vi "Begin.vi"() -> (0 "error out 2":errorcluster)   [LabVIEW 2014]
doc: "Called before other user functions, this VI is expected to open initial I/O refnums, load in file data, and do all program initialization. Notice that the <B>error out</B> terminal is simply used for data flow. Wiring it to other structures or subVIs ensures that this VI runs first."
uses:
  <vilib>/Rock Robotics/WPI/SafetyOutput/WPI_SafetyOutputConfigMenu.ctl
  <vilib>/Rock Robotics/WPI/DriverStation/WPI_DriverStationRobotMode2.ctl
  <vilib>/Rock Robotics/SystemInterfaces/DIO/FPGA_DIOPWMChannel.ctl
  <vilib>/Rock Robotics/WPI/Joystick/WPI_JoystickDeviceEnum.ctl
  <vilib>/Rock Robotics/SystemInterfaces/DIO/FPGA_DIOChannel.ctl
  <vilib>/Rock Robotics/SystemInterfaces/AI/FPGA_AIGyroChannel.ctl
  <vilib>/Rock Robotics/SystemInterfaces/Typedef/FPGA_TypedefAnalogModuleForGyro.ctl
  <vilib>/Rock Robotics/WPI/Solenoid/WPI_SolenoidChannel.ctl
  <vilib>/Rock Robotics/SystemInterfaces/Typedef/FPGA_TypedefDigitalModule.ctl
  <vilib>/Rock Robotics/SystemInterfaces/AI/FPGA_AIChannel.ctl
  <vilib>/Rock Robotics/SystemInterfaces/Typedef/FPGA_TypedefAnalogModule.ctl
  <vilib>/Rock Robotics/SystemInterfaces/DIO/FPGA_DIORelayChannel.ctl
  Robot Global Data.vi
  <vilib>/Rock Robotics/WPI/RobotDrive/WPI_RobotDriveOpen4MotorWithTalon.vi
  <vilib>/Rock Robotics/Network Tables/SD Write String Array.vi
  <vilib>/Rock Robotics/WPI/Counter/WPI_CounterDigitalInputToDigitalSource.vi
  <vilib>/Rock Robotics/WPI/Solenoid/WPI_SolenoidOpenDouble.vi
  <vilib>/Rock Robotics/WPI/Solenoid/WPI_SolenoidOpenSingle.vi
  <vilib>/Rock Robotics/WPI/MotorControl/WPI_MotorControlOpen Talon.vi
  TORC Code/GlobalVariable.vi
  Moose Code/Auto_Conf.vi
  <vilib>/Rock Robotics/WPI/Compressor/WPI_CompressorGetSetRefNum.vi
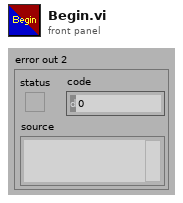
[diagram p1: front panel]
types:
  T1 = typedef "WPI_JoystickDeviceEnum.ctl" = enum16{"USB 0", "USB 1", "USB 2", "USB 3", "USB 4", "USB 5"}
  T2 = typedef "FPGA_DIORelayChannel.ctl" = enum8{"Relay 0", "Relay 1", "Relay 2", "Relay 3", "Invalid"}
  T3 = typedef "FPGA_DIOChannel.ctl" = enum8{"DIO 0", "DIO 1", "DIO 2", "DIO 3", "DIO 4", "DIO 5", "DIO 6", "DIO 7", "DIO 8", "DIO 9", "DIO MXP 0", "DIO MXP 1", "DIO MXP 2", "DIO MXP 3", "DIO MXP 4", "DIO MXP 5", "DIO MXP 6", "DIO MXP 7", "DIO MXP 8", "DIO MXP 9", "DIO MXP 10", "DIO MXP 11", "DIO MXP 12", "DIO MXP 13", "DIO MXP 14", "DIO MXP 15", "Invalid"}
  T4 = typedef "FPGA_TypedefAnalogModule.ctl" = enum16{"Controller 1"}
  T5 = typedef "FPGA_AIChannel.ctl" = enum8{"AI 0", "AI 1", "AI 2", "AI 3", "AI MXP 0", "AI MXP 1", "AI MXP 2", "AI MXP 3", "Invalid"}
  T6 = typedef "FPGA_DIOPWMChannel.ctl" = enum8{"PWM 0", "PWM 1", "PWM 2", "PWM 3", "PWM 4", "PWM 5", "PWM 6", "PWM 7", "PWM 8", "PWM 9", "PWM MXP 0", "PWM MXP 1", "PWM MXP 2", "PWM MXP 3", "PWM MXP 4", "PWM MXP 5", "PWM MXP 6", "PWM MXP 7", "PWM MXP 8", "PWM MXP 9", "Invalid"}
  T7 = typedef "FPGA_TypedefDigitalModule.ctl" = enum16{"Controller 1"}
  T8 = typedef "WPI_SolenoidChannel.ctl" = enum8{"Solenoid 0", "Solenoid 1", "Solenoid 2", "Solenoid 3", "Solenoid 4", "Solenoid 5", "Solenoid 6", "Solenoid 7", "Invalid"}
  T9 = typedef "FPGA_TypedefAnalogModuleForGyro.ctl" = enum16{"Controller 1"}
  T10 = typedef "FPGA_AIGyroChannel.ctl" = enum8{"AI 0", "AI 1", "Invalid"}
  T11 = typedef "WPI_DriverStationRobotMode2.ctl" = enum16{"Autonomous Disabled", "Autonomous Enabled", "Teleop Disabled", "Teleop Enabled", "Disconnected", "Finish", "Test Disabled", "Test Enabled", "Emergency Stopped"}
  T12 = typedef "WPI_SafetyOutputConfigMenu.ctl" = enum16{"Enable", "Disable"}
  T13 = typedef "WPI_JoystickDevRef.ctl" = cluster{"Device":T1}
  T14 = typedef "WPI_DigitalInputDevRef.ctl" = cluster{"DevStatus":errorcluster, "DIO Channel":T3, "Controller":T7}
  T15 = typedef "WPI_SolenoidDevRef.ctl" = cluster{"DevStatus":errorcluster, "Pneumatics Control Module":u8, "Forward Solenoid Channel":T8, "Reverse Solenoid Channel":T8}
  T16 = typedef "FPGA_CounterEncoderSourceConvertionLVSourceType.ctl" = cluster{"DevStatus":errorcluster, "AnalogTriggerMode?":bool, "DigitalMode":cluster{"Controller":T7, "DIO Channel":T17}, "AnalogTriggerMode":cluster{"AnalogTriggerIndex":T18, "OutputType":T19}}
  T17 = typedef "FPGA_DIODigitalSourceChannel.ctl" = enum8{"DIO 0", "DIO 1", "DIO 2", "DIO 3", "DIO 4", "DIO 5", "DIO 6", "DIO 7", "DIO 8", "DIO 9", "DIO MXP 0", "DIO MXP 1", "DIO MXP 2", "DIO MXP 3", "DIO MXP 4", "DIO MXP 5", "DIO MXP 6", "DIO MXP 7", "DIO MXP 8", "DIO MXP 9", "DIO MXP 10", "DIO MXP 11", "DIO MXP 12", "DIO MXP 13", "DIO MXP 14", "DIO MXP 15", "Disabled"}
  T18 = typedef "FPGA_AnalogTriggerIndex.ctl" = enum8{"Trig 0", "Trig 1", "Trig 2", "Trig 3", "Trig 4", "Trig 5", "Trig 6", "Trig 7", "Invalid"}
  T19 = typedef "FPGA_AnalogTriggerOutType.ctl" = enum16{"InWindow", "TriggerState", "Rising", "Falling"}
  T20 = typedef "WPI_RobotDriveDevRef.ctl" = cluster{"DevStatus":errorcluster, "Motors[]":T21[], "Square Inputs":bool, "Max Output":dbl}
  T21 = typedef "WPI_MotorControlDeviceRef.ctl" = cluster{"DeviceStatus":errorcluster, "Type":T22, "PWM":cluster{"Controller":T7, "PWM Channel":T6, "DeadBand":T23}, "CAN":cluster{"Device Number":u8, "Control Mode":T24, "Semaphore":T25, "Max Vout":dbl, "TalonSRX Control Mode":T26}, "Invert":bool, "TransformRef":T27, "InvTransformRef":T27}
  T22 = typedef "WPI_MotorControlType.ctl" = enum16{"PWM", "CAN", "CANTalonSRX"}
  T23 = typedef "WPI_PWMDeadband.ctl" = cluster{"Name":string, "maxPositivePwm":i32, "minPositivePwm":i32, "centerPwm":i32, "maxNegativePwm":i32, "minNegativePwm":i32, "angularRange":u16}
  T24 = typedef "WPI_CANJaguar_ControlMode.ctl" = enum8{"Percent VBus", "Current", "Speed", "Position", "Voltage"}
  T25 = typedef "Semaphore RefNum" = refnum<k1>
  T26 = typedef "WPI_CANTalonSRX_APIControlMode.ctl" = enum8{"Percent VBus", "Speed", "Position", "Slave", "Unchanged / Invalid"}
  T27 = typedef "WPI_PWMTransform_ConPane.ctl" = refnum<vi>
  T28 = typedef "WPI_EncoderDevRef.ctl" = cluster{"DevStatus":errorcluster, "EncoderIndex":T29, "CounterIndex":T30, "DistancePerCount":dbl, "Decoding Type":T31}
  T29 = typedef "FPGA_EncoderIdx.ctl" = enum8{"Enc 0", "Enc 1", "Enc 2", "Enc 3", "Enc 4", "Enc 5", "Enc 6", "Enc 7", "Invalid"}
  T30 = typedef "FPGA_CounterCtrSystemIndex.ctl" = enum8{"Ctr 0", "Ctr 1", "Ctr 2", "Ctr 3", "Ctr 4", "Ctr 5", "Ctr 6", "Ctr 7", "Invalid"}
  T31 = typedef "WPI_EncoderType.ctl" = enum16{"1x", "2x", "4x"}
  T32 = typedef "WPI_CompressorDevRef.ctl" = cluster{"DevStatus":errorcluster, "Pneumatics Control Module":u8}
  T33 = typedef "WPI_AnalogChannelDevRef.ctl" = cluster{"DevStatus":errorcluster, "Controller":T4, "Analog Channel":T5}
  T34 = typedef "WPI_RelayDevRef.ctl" = cluster{"DevStatus":errorcluster, "Relay Channel":T2, "Controller":T7, "Relay Direction":T35}
  T35 = typedef "WPI_RelayDirection.ctl" = enum16{"Both directions", "Forward only", "Reverse only"}
  T36 = typedef "WPI_GyroDevRef.ctl" = cluster{"DevStatus":errorcluster, "Analog Module":T4, "Analog Channel":T5, "Offset":dbl, "Gain (VoltsPerDegree/Second)":dbl}
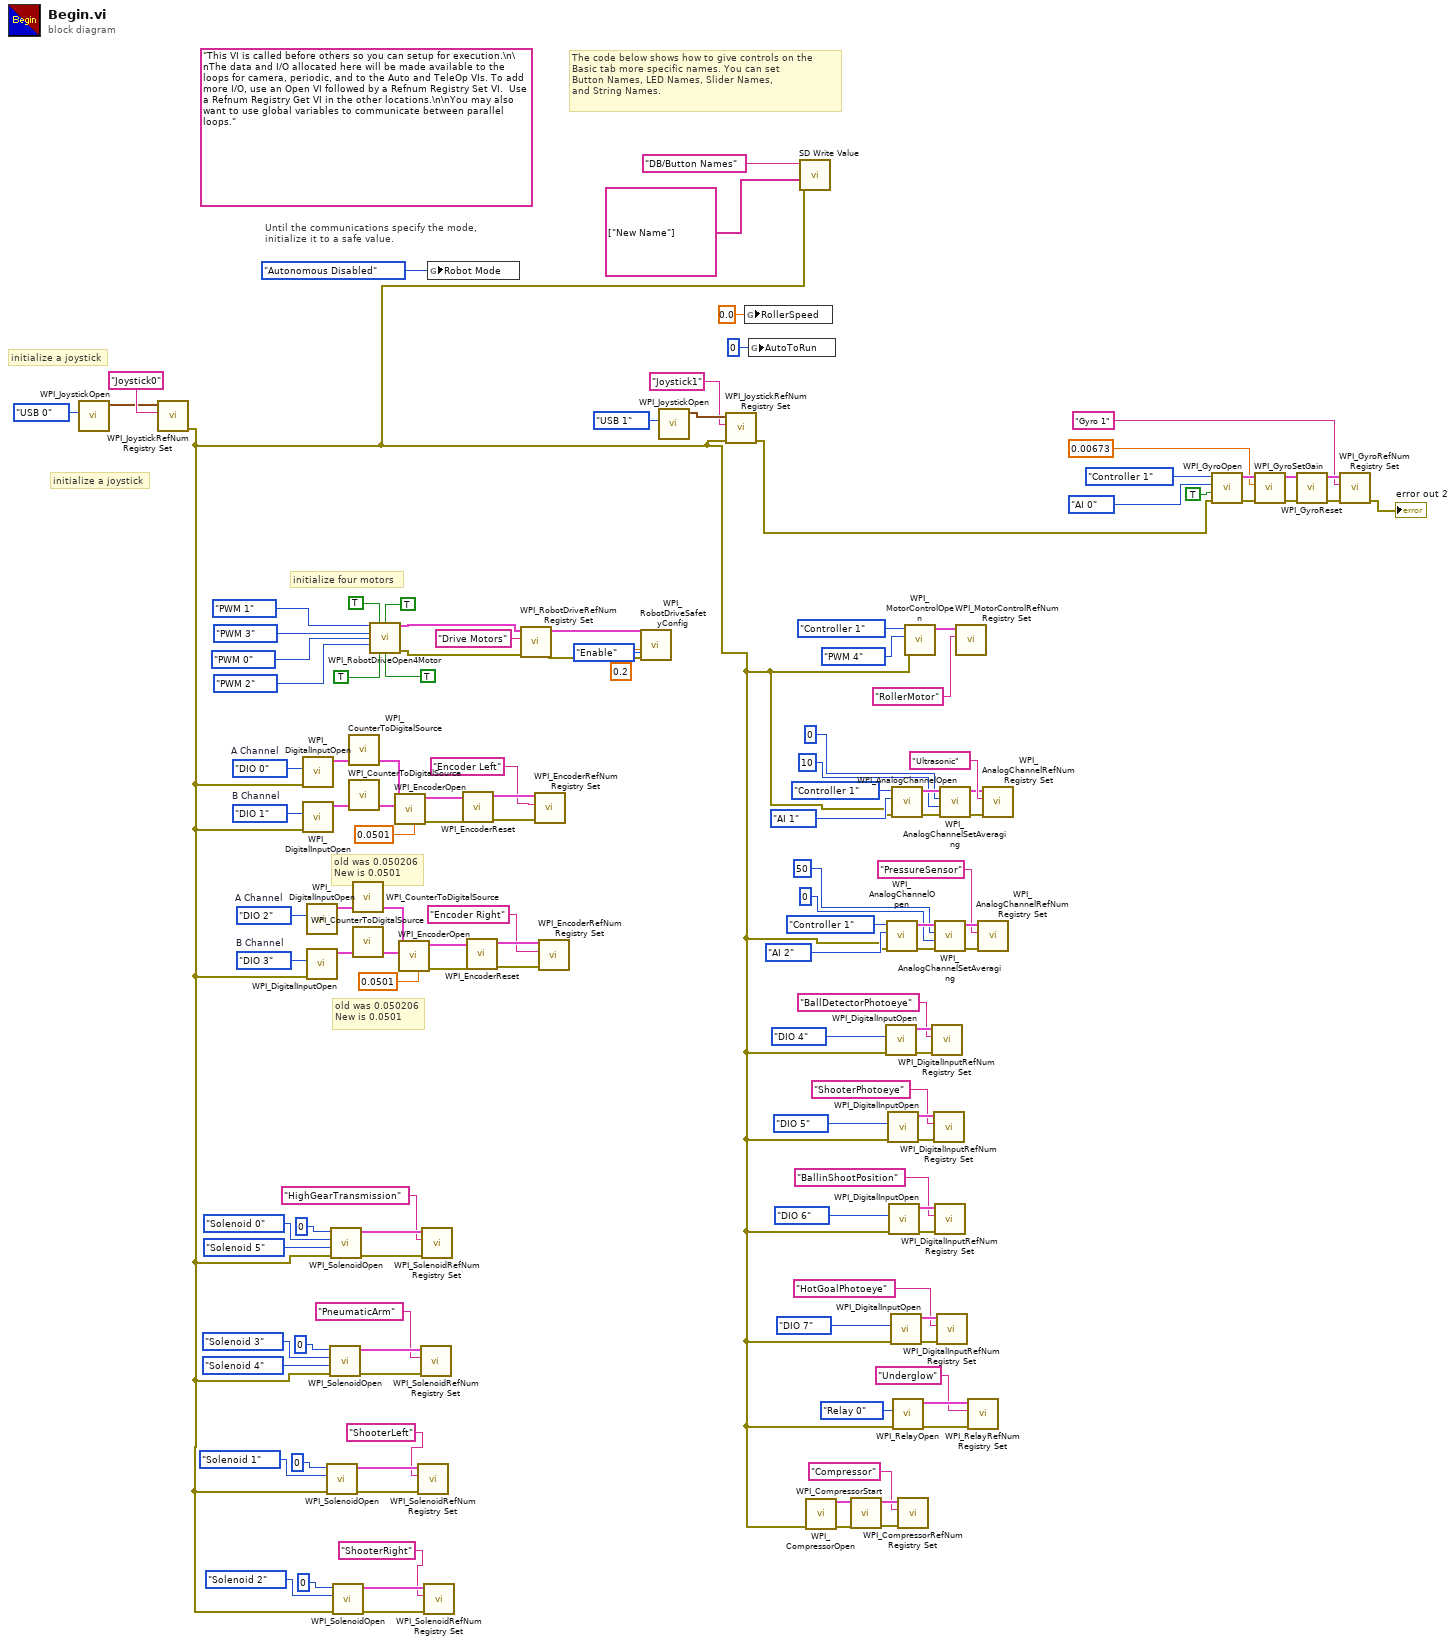
[diagram p0: block diagram]
diagram:
  w102 = FPGA_DIOChannel."DIO 1"  # B Channel
  w101 = FPGA_DIOChannel."DIO 0"  # A Channel
  w114 = FPGA_DIOChannel."DIO 3"  # B Channel
  w113 = FPGA_DIOChannel."DIO 2"  # A Channel
  (unwired) "This VI is called before others so you can setup for execution.\n\nThe data and I/O allocated here will be made available to the loops for camera, periodic, and to the Auto and TeleOp VIs. To add more I/O, use an Open VI followed by a Refnum Registry Set VI.  Use a Refnum Registry Get VI in the other locations.\n\nYou may also want to use global variables to communicate between parallel loops."
  # "old was 0.050206\nNew is 0.0501"
  # "old was 0.050206\nNew is 0.0501"
  # "initialize a joystick"
  # "The code below shows how to give controls on the\nBasic tab more specific names. You can set\nButton Names, LED Names, Slider Names,\nand String Names."
  # "initialize a joystick"
  # "Until the communications specify the mode,\ninitialize it to a safe value."
  # "initialize four motors"
  n1 = call <vilib>:"WPI_JoystickOpen.vi"("JoystickDevice"=WPI_JoystickDeviceEnum."USB 0") -> ("JoystickDevRef"=w116:T13)  [unwired: 10 in]
  n2 = call <vilib>:"WPI_JoystickRefNum Registry Set.vi"("refnum name"="Joystick0", "JoystickDevRef"=w116) -> ("error out"=w1:errorcluster)  [unwired: 8 in, 1 out]
  n3 = call <vilib>:"WPI_DigitalInputOpen.vi"("error in (no error)"=w1, "DIO Channel"=w101) -> ("DigitalInputDevRef"=w98:T14)  [unwired: 1 in, 8 out]
  n4 = call <vilib>:"WPI_DigitalInputOpen.vi"("error in (no error)"=w1, "DIO Channel"=w102) -> ("DigitalInputDevRef"=w99:T14)  [unwired: 1 in, 8 out]
  n5 = call <vilib>:"WPI_DigitalInputOpen.vi"("DIO Channel"=w113) -> ("DigitalInputDevRef"=w110:T14)  [unwired: 2 in, 8 out]
  n6 = call <vilib>:"WPI_DigitalInputOpen.vi"("error in (no error)"=w1, "DIO Channel"=w114) -> ("DigitalInputDevRef"=w111:T14)  [unwired: 1 in, 8 out]
  n7 = call-poly <vilib>:"WPI_SolenoidOpen.vi"("error in (no error)"=w1, "Solenoid Channel"=WPI_SolenoidChannel."Solenoid 1" ("Forward Solenoid Channel"), "Pneumatics Control Module (0)"=u8 0) -> ("error out"=w66:errorcluster, "SolenoidDevRef"=w65:T15)  [unwired: 7 in]
  n8 = call-poly <vilib>:"WPI_SolenoidOpen.vi"("error in (no error)"=w1, "Reverse Solenoid Channel"=WPI_SolenoidChannel."Solenoid 4", "Forward Solenoid Channel"=WPI_SolenoidChannel."Solenoid 3", "Pneumatics Control Module (0)"=u8 0) -> ("error out"=w70:errorcluster, "SolenoidDevRef"=w69:T15)  [unwired: 6 in]
  n9 = call-poly <vilib>:"WPI_SolenoidOpen.vi"("error in (no error)"=w1, "Reverse Solenoid Channel"=WPI_SolenoidChannel."Solenoid 5", "Forward Solenoid Channel"=WPI_SolenoidChannel."Solenoid 0", "Pneumatics Control Module (0)"=u8 0) -> ("error out"=w76:errorcluster, "SolenoidDevRef"=w75:T15)  [unwired: 6 in]
  n10 = call-poly <vilib>:"WPI_SolenoidOpen.vi"("error in (no error)"=w1, "Solenoid Channel"=WPI_SolenoidChannel."Solenoid 2" ("Forward Solenoid Channel"), "Pneumatics Control Module (0)"=u8 0) -> ("error out"=w62:errorcluster, "SolenoidDevRef"=w61:T15)  [unwired: 7 in]
  n11 = call-poly <vilib>:"WPI_CounterToDigitalSource.vi"("DigitalInputDevRef"=w98) -> ("Digital Source"=w97:T16)  [unwired: 6 out]
  n12 = call-poly <vilib>:"WPI_CounterToDigitalSource.vi"("DigitalInputDevRef"=w99) -> ("Digital Source"=w100:T16)  [unwired: 6 out]
  n13 = call-poly <vilib>:"WPI_CounterToDigitalSource.vi"("DigitalInputDevRef"=w110) -> ("Digital Source"=w109:T16)  [unwired: 6 out]
  n14 = call-poly <vilib>:"WPI_CounterToDigitalSource.vi"("DigitalInputDevRef"=w111) -> ("Digital Source"=w112:T16)  [unwired: 6 out]
  n15 = call-poly <vilib>:"WPI_RobotDriveOpen4Motor.vi"("Rear Left Motor"=FPGA_DIOPWMChannel."PWM 1", "Rear Left Motor Inverted"=TRUE, "Rear Right Motor Inverted"=TRUE, "Rear Right Motor"=FPGA_DIOPWMChannel."PWM 3", "Front Left Motor"=FPGA_DIOPWMChannel."PWM 0", "Front Right Motor"=FPGA_DIOPWMChannel."PWM 2", "Front Left Motor Inverted"=TRUE, "Front Right Motor Inverted"=TRUE) -> ("RobotDriveDevRef"=w127:T20, "error out"=w118:errorcluster)  [unwired: 6 in]
  n16 = call <vilib>:"WPI_EncoderOpen.vi"("DistancePerCount"=0.0501, "BSource"=w100, "ASource"=w97) -> ("error out"=w93:errorcluster, "EncoderDevRef"=w96:T28)  [unwired: 5 in, 2 out]
  n17 = call <vilib>:"WPI_EncoderOpen.vi"("DistancePerCount"=0.0501, "BSource"=w112, "ASource"=w109) -> ("error out"=w104:errorcluster, "EncoderDevRef"=w108:T28)  [unwired: 5 in, 2 out]
  n18 = call <vilib>:"WPI_SolenoidRefNum Registry Set.vi"("error in (no error)"=w66, "refnum name"="ShooterLeft", "SolenoidDevRef"=w65) -> ()  [unwired: 7 in, 2 out]
  n19 = call <vilib>:"WPI_SolenoidRefNum Registry Set.vi"("error in (no error)"=w70, "refnum name"="PneumaticArm", "SolenoidDevRef"=w69) -> ()  [unwired: 7 in, 2 out]
  n20 = call <vilib>:"WPI_SolenoidRefNum Registry Set.vi"("error in (no error)"=w76, "refnum name"="HighGearTransmission", "SolenoidDevRef"=w75) -> ()  [unwired: 7 in, 2 out]
  n21 = call <vilib>:"WPI_SolenoidRefNum Registry Set.vi"("error in (no error)"=w62, "refnum name"="ShooterRight", "SolenoidDevRef"=w61) -> ()  [unwired: 7 in, 2 out]
  n22 = global write "Robot Global Data.vi" "Robot Mode"(WPI_DriverStationRobotMode2."Autonomous Disabled" ("Robot Mode")) -> ()
  n23 = call <vilib>:"WPI_EncoderReset.vi"("error in (no error)"=w93, "EncoderDevRef"=w96) -> ("error out"=w92:errorcluster, "EncoderDevRef"=w95:T28)  [unwired: 8 in]
  n24 = call <vilib>:"WPI_EncoderReset.vi"("error in (no error)"=w104, "EncoderDevRef"=w108) -> ("error out"=w103:errorcluster, "EncoderDevRef"=w107:T28)  [unwired: 8 in]
  n25 = call <vilib>:"WPI_RobotDriveRefNum Registry Set.vi"("error in (no error)"=w118, "refnum name"="Drive Motors", "RobotDriveDevRef"=w127) -> ("error out"=w5:errorcluster, "RobotDriveDevRef"=w129:T20)  [unwired: 7 in]
  n26 = call <vilib>:"WPI_EncoderRefNum Registry Set.vi"("error in (no error)"=w92, "refnum name"="Encoder Left", "EncoderDevRef"=w95) -> ()  [unwired: 7 in, 2 out]
  n27 = call <vilib>:"WPI_EncoderRefNum Registry Set.vi"("error in (no error)"=w103, "refnum name"="Encoder Right", "EncoderDevRef"=w107) -> ()  [unwired: 7 in, 2 out]
  n28 = call <vilib>:"WPI_RobotDriveSafetyConfig.vi"("error in (no error)"=w5, "timeout (s)"=0.2, "mode"=WPI_SafetyOutputConfigMenu."Enable", "RobotDriveDevRef"=w129) -> ()  [unwired: 6 in, 2 out]
  n29 = call <vilib>:"WPI_JoystickOpen.vi"("JoystickDevice"=WPI_JoystickDeviceEnum."USB 1") -> ("JoystickDevRef"=w8:T13)  [unwired: 10 in]
  n30 = call <vilib>:"WPI_JoystickRefNum Registry Set.vi"("error in (no error)"=w1, "refnum name"="Joystick1", "JoystickDevRef"=w8) -> ("error out"=w2:errorcluster)  [unwired: 7 in, 1 out]
  n31 = global write "GlobalVariable.vi" "RollerSpeed"(0.0 ("RollerSpeed")) -> ()
  n32 = global write "Auto_Conf.vi" "AutoToRun"(u8 0 ("AutoToRun")) -> ()
  n33 = call-poly <vilib>:"SD Write Value.vi"("error in"=w1, "String Array"=string[] ["New Name"], "Name"="DB/Button Names") -> ()  [unwired: 7 in, 2 out]
  n34 = call <vilib>:"WPI_CompressorOpen.vi"("error in (no error)"=w1) -> ("CompressorDevRef"=w12:T32, "error out"=w13:errorcluster)  [unwired: 13 in]
  n35 = call <vilib>:"WPI_CompressorStart.vi"("error in (no error)"=w13, "CompressorDevRef"=w12) -> ("error out"=w11:errorcluster, "CompressorDevRef"=w10:T32)  [unwired: 8 in]
  n36 = call <vilib>:"WPI_DigitalInputOpen.vi"("error in (no error)"=w1, "DIO Channel"=FPGA_DIOChannel."DIO 4") -> ("error out"=w32:errorcluster, "DigitalInputDevRef"=w34:T14)  [unwired: 8 in]
  n37 = call <vilib>:"WPI_AnalogChannelOpen.vi"("error in (no error)"=w1, "Analog Channel"=FPGA_AIChannel."AI 2", "Controller"=FPGA_TypedefAnalogModule."Controller 1") -> ("error out"=w50:errorcluster, "AIDeviceRef"=w51:T33)  [unwired: 7 in]
  n38 = call <vilib>:"WPI_DigitalInputOpen.vi"("error in (no error)"=w1, "DIO Channel"=FPGA_DIOChannel."DIO 5") -> ("error out"=w29:errorcluster, "DigitalInputDevRef"=w30:T14)  [unwired: 8 in]
  n39 = call <vilib>:"WPI_DigitalInputOpen.vi"("error in (no error)"=w1, "DIO Channel"=FPGA_DIOChannel."DIO 6") -> ("error out"=w26:errorcluster, "DigitalInputDevRef"=w27:T14)  [unwired: 8 in]
  n40 = call <vilib>:"WPI_DigitalInputOpen.vi"("error in (no error)"=w1, "DIO Channel"=FPGA_DIOChannel."DIO 7") -> ("error out"=w23:errorcluster, "DigitalInputDevRef"=w24:T14)  [unwired: 8 in]
  n41 = call <vilib>:"WPI_AnalogChannelOpen.vi"("error in (no error)"=w1, "Analog Channel"=FPGA_AIChannel."AI 1", "Controller"=FPGA_TypedefAnalogModule."Controller 1") -> ("error out"=w41:errorcluster, "AIDeviceRef"=w42:T33)  [unwired: 7 in]
  n42 = call <vilib>:"WPI_RelayOpen.vi"("error in (no error)"=w1, "Relay Channel"=FPGA_DIORelayChannel."Relay 0") -> ("error out"=w18:errorcluster, "RelayDevRef"=w19:T34)  [unwired: 8 in]
  n43 = call <vilib>:"WPI_CompressorRefNum Registry Set.vi"("error in (no error)"=w11, "refnum name"="Compressor", "CompressorDevRef"=w10) -> ()  [unwired: 7 in, 2 out]
  n44 = call-poly <vilib>:"WPI_MotorControlOpen.vi"("error in (no error)"=w1, "PWM Channel"=FPGA_DIOPWMChannel."PWM 4", "Controller"=FPGA_TypedefDigitalModule."Controller 1") -> ("MotorControlDeviceRef"=w57:T21)  [unwired: 7 in, 1 out]
  n45 = call <vilib>:"WPI_DigitalInputRefNum Registry Set.vi"("error in (no error)"=w32, "refnum name"="BallDetectorPhotoeye", "DigitalInputDevRef"=w34) -> ()  [unwired: 7 in, 2 out]
  n46 = call <vilib>:"WPI_DigitalInputRefNum Registry Set.vi"("error in (no error)"=w29, "refnum name"="ShooterPhotoeye", "DigitalInputDevRef"=w30) -> ()  [unwired: 7 in, 2 out]
  n47 = call <vilib>:"WPI_AnalogChannelSetAveraging.vi"("error in (no error)"=w50, "OversampleBits"=u8 0, "AverageBits"=u8 50, "AIDeviceRef"=w51) -> ("error out"=w49:errorcluster, "AIDeviceRef"=w52:T33)  [unwired: 6 in]
  n48 = call <vilib>:"WPI_DigitalInputRefNum Registry Set.vi"("error in (no error)"=w26, "refnum name"="BallinShootPosition", "DigitalInputDevRef"=w27) -> ()  [unwired: 7 in, 2 out]
  n49 = call <vilib>:"WPI_DigitalInputRefNum Registry Set.vi"("error in (no error)"=w23, "refnum name"="HotGoalPhotoeye", "DigitalInputDevRef"=w24) -> ()  [unwired: 7 in, 2 out]
  n50 = call <vilib>:"WPI_AnalogChannelSetAveraging.vi"("error in (no error)"=w41, "OversampleBits"=u8 10, "AverageBits"=u8 0, "AIDeviceRef"=w42) -> ("error out"=w40:errorcluster, "AIDeviceRef"=w43:T33)  [unwired: 6 in]
  n51 = call <vilib>:"WPI_MotorControlRefNum Registry Set.vi"("refnum name"="RollerMotor", "MotorControlDevRef"=w57) -> ()  [unwired: 8 in, 2 out]
  n52 = call <vilib>:"WPI_RelayRefNum Registry Set.vi"("error in (no error)"=w18, "refnum name"="Underglow", "RelayDevRef"=w19) -> ()  [unwired: 7 in, 2 out]
  n53 = call <vilib>:"WPI_AnalogChannelRefNum Registry Set.vi"("error in (no error)"=w49, "refnum name"="PressureSensor", "AIDeviceRef"=w52) -> ()  [unwired: 7 in, 2 out]
  n54 = call <vilib>:"WPI_AnalogChannelRefNum Registry Set.vi"("error in (no error)"=w40, "refnum name"="Ultrasonic", "AIDeviceRef"=w43) -> ()  [unwired: 7 in, 2 out]
  n55 = call <vilib>:"WPI_GyroOpen.vi"("error in (no error)"=w2, "Calibrate On Open"=TRUE, "Analog Channel"=FPGA_AIGyroChannel."AI 0", "Controller"=FPGA_TypedefAnalogModuleForGyro."Controller 1") -> ("error out"=w90:errorcluster, "GyroDevRef"=w89:T36)  [unwired: 5 in, 1 out]
  n56 = call <vilib>:"WPI_GyroSetGain.vi"("error in (no error)"=w90, "Gain (VoltsPerDegree/Second)"=0.00673, "GyroDevRef"=w89) -> ("error out"=w88:errorcluster, "GyroDevRef"=w87:T36)  [unwired: 7 in]
  n57 = call <vilib>:"WPI_GyroReset.vi"("error in (no error)"=w88, "GyroDevRef"=w87) -> ("error out"=w86:errorcluster, "GyroDevRef"=w85:T36)  [unwired: 8 in]
  n58 = call <vilib>:"WPI_GyroRefNum Registry Set.vi"("error in (no error)"=w86, "refnum name"="Gyro 1", "GyroDevRef"=w85) -> ("error out"=→"error out 2":errorcluster)  [unwired: 7 in, 1 out]
